vi "Create Pressure Task.vi"(8 "error in":errorcluster, 11 "physical channel":string="cDAQ3Mod1/ai0") -> (0 "error out":errorcluster, 3 "task out":refnum<k21>)   [LabVIEW 2013]
uses:
  <vilib>/DAQmx/create/channels.llb/DAQmx Create Channel (AI-Current-Basic).vi
  <resource>/objmgr/daqmx.rc
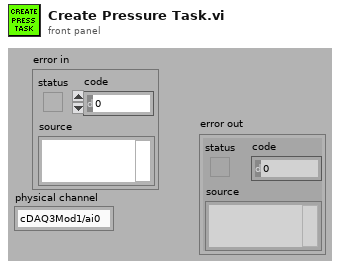
[diagram p1: front panel]
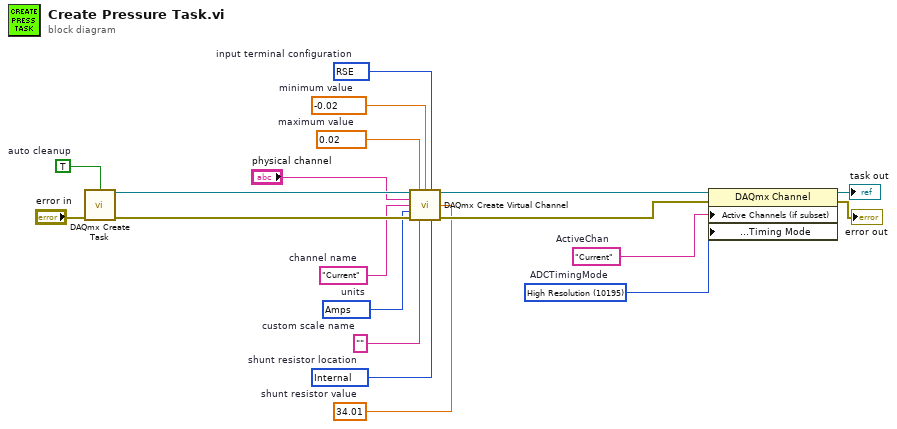
[diagram p0: block diagram]
diagram:
  w2 = 10195 items=["High Resolution"=10195, "High Speed"=14712, "Best 50 Hz Rejection"=14713, "Best 60 Hz Rejection"=14714]  # ADCTimingMode
  w5 = "Current"  # ActiveChan
  w6 = 10083 items=["default"=-1, "RSE"=10083, "NRSE"=10078, "Differential"=10106, "Pseudodifferential"=12529]  # input terminal configuration
  w7 = 10342 items=["Amps"=10342, "From Custom Scale"=10065]  # units
  w8 = 34.01  # shunt resistor value
  w9 = 10200 items=["Internal"=10200, "External"=10167]  # shunt resistor location
  w10 = "Current"  # channel name
  w12 = ""  # custom scale name
  w13 = -0.02  # minimum value
  w14 = 0.02  # maximum value
  w17 = TRUE  # auto cleanup
  n1 = call <vilib>:"DAQmx Create Task.vi"("auto cleanup"=w17, "error in"="error in") -> ("task out"=w16:refnum<k21>, "error out"=w18:errorcluster)  [unwired: 12 in]
  n2 = call-poly <vilib>:"DAQmx Create Virtual Channel.vi"("task in"=w16, "maximum value"=w14, "minimum value"=w13, "input terminal configuration"=w6, "physical channels"="physical channel", "name to assign"=w10, "external shunt resistor value"=w8, "units"=w7, "error in"=w18, "custom scale name"=w12, "shunt resistor location"=w9) -> ("task out"=w1:refnum<k21>, "error out"=w11:errorcluster)  [unwired: 3 in]
  n3 = property class="DAQmx Channel"(reference=w1, error in=w11, "Active Channels (if subset)"=w5, "Analog Input:General Properties:Digitizer/ADC:Timing Mode"=w2) -> (reference out=→"task out":refnum<k21>, error out=→"error out":errorcluster)
